vi "One Cycle Delay.vi"(8 "error in (no error)":errorcluster) -> (0 "error out":errorcluster)   [LabVIEW 2016, in "IgusMotorDrive.lvclass"]
uses:
  IgusMotorDrive.lvclass
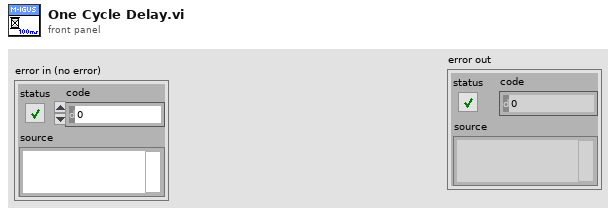
[diagram p1: front panel]
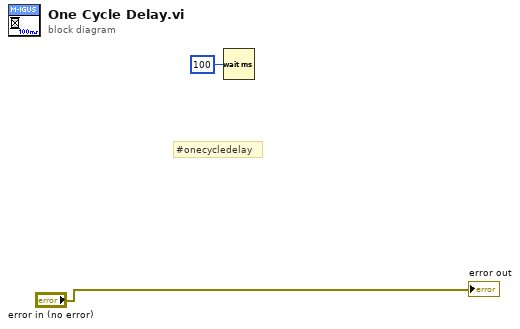
[diagram p0: block diagram]
diagram:
  # "#onecycledelay"
  n1 = Wait (ms)(milliseconds to wait=u32 100) -> ()  [unwired: 1 out]
  "error out" <- "error in (no error)"
